vi "TCL Select Current Fragments 1frag1criterium.vi"(3 "error in (no error)":errorcluster, 4 "criterium":T1={"fragment"="", "values"=[], "operator"="is equal to"}, 5 "fragment":string) -> (0 "error out":errorcluster, 1 "matches":string[][](array[string]), 2 "fragments out":string[](array[string]))   [LabVIEW 2010]
uses:
  TCL Global.vi
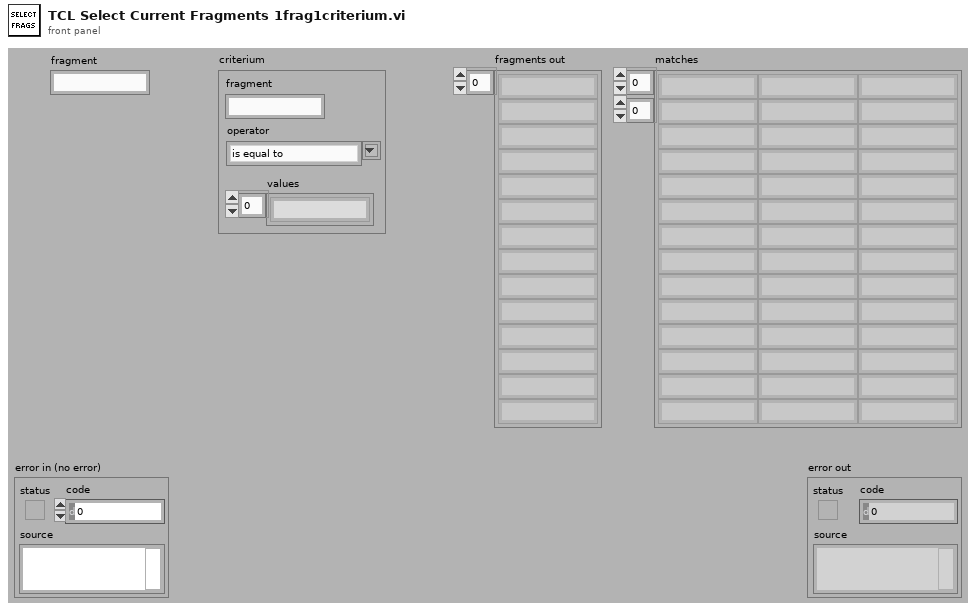
[diagram p1: front panel]
types:
  T1 = cluster{"fragment":string, "values":string[], "operator":string}
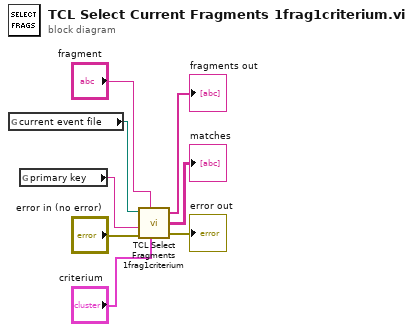
[diagram p0: block diagram]
diagram:
  n1 = global read "TCL Global.vi" "current event file"() -> (w2:path)
  n2 = global read "TCL Global.vi" "primary key"() -> (w1:string)
  n3 = call "TCL Select Fragments 1frag1criterium.vi"("event file"=w2, "fragment"="fragment", "primary key"=w1, "criterium"="criterium", "error in (no error)"="error in (no error)") -> ("fragments out"=→"fragments out":string[], "matches"=→"matches":string[][], "error out"=→"error out":errorcluster)  [unwired: 1 in]
